vi "WriteToInstrument.vi"(2 "New values":cluster{"Inst #":string, "Value":dbl}[](array[cluster]), 3 "Inst. array in":cluster{"Inst #":string, "Value":dbl}[](array[cluster])) -> (1 "Inst. array out":cluster{"Inst #":string, "Value":dbl}[](array[cluster]))   [LabVIEW 2020]
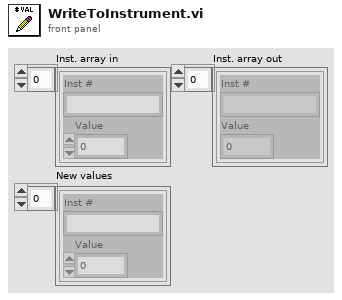
[diagram p1: front panel]
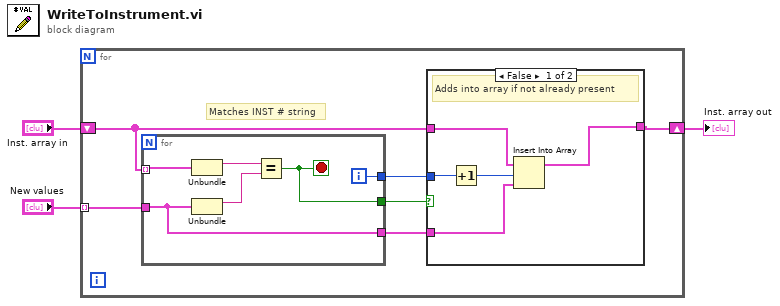
[diagram p0: block diagram]
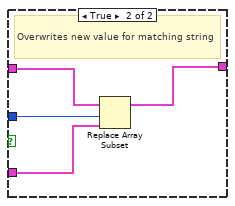
[diagram p2: hidden frame]
diagram:
  n1 = for {
    tunnel: "New values" -> [w4] mode=indexing
    shift-right: [w8] -> w2
    shift-left: "Inst. array in" -> [w9]
    # "Matches INST # string"
    n2 = for {
      tunnel: w4 -> [w21]
      tunnel: w9 -> [w22] mode=indexing
      tunnel: [w21] -> w7
      tunnel: [w20] -> w6
      tunnel: [w19] -> w5
      i -> [w20]
      stop <- w19 stop-if-true
      n3 = Unbundle(w22) -> ("Inst #"=w24:string)  [unwired: 1 out]
      n4 = Unbundle(w21) -> ("Inst #"=w23:string)  [unwired: 1 out]
      n5 = Equal?(x=w24, y=w23) -> (x = y?=w19:bool)
    }
    n6 = case shown="False" w5 {
      tunnel: w9 -> [w12 w18]
      tunnel: w7 -> [w14 w17]
      tunnel: w6 -> [w11 w16]
      tunnel: [w13 w15] -> w8
      frame False {
        # "Adds into array if not already present"
        n7 = Increment(x=w11) -> (x+1=w10:i32)
        n8 = Insert Into Array(array=w12, index=w10, new element=w14) -> (w13:cluster{"Inst #":string, "Value":dbl}[])
      }
      frame True {
        # "Overwrites new value for matching string"
        n9 = Replace Array Subset(array=w18, new element=w17, index=w16) -> (w15:cluster{"Inst #":string, "Value":dbl}[])
      }
    }
  }
  "Inst. array out" <- w2
